vi "LakeShore 370 curve.vi"(2 "error in (no error)":errorcluster, 3 "Curve Data Format 1: Log Ohms/K)":u16(ring)=1 items=["Ohms/K", "Log Ohms/K"], 4 "Curve (1)":i32=1 min=1 max=20 step=1, 5 "VISA session":refnum<visa-resource-name>) -> (0 "error out":errorcluster, 1 "dup VISA session":refnum<visa-resource-name>)   [LabVIEW 2019]
doc: "This VI will upload a calibration curve to the LakeShore 370 AC Resistance Bridge. It reads the data from a file and then formats it for uploading.\nScott Hannahs, <sth@magnet.fsu.edu> NHMFL-FSU, May 2003"
uses:
  Misc Extras/Manufacturer Drivers/LakeShore/Lake Shore Cryotronics 370/Lake Shore Cryotronics 370.lvlib
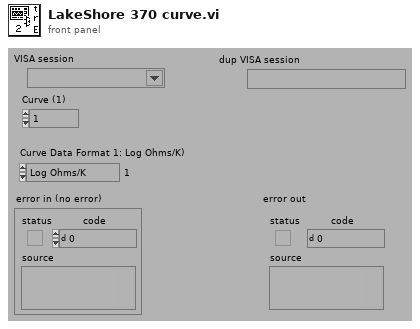
[diagram p1: front panel]
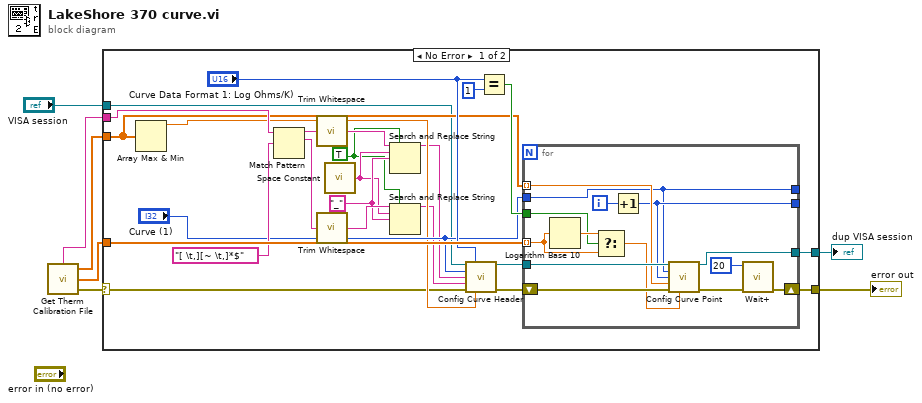
[diagram p0: block diagram]
diagram:
  n1 = call "Get Therm Calibration File.vi"() -> ("Calbration Name"=w6:string, "Temperature"=w5:dbl[], "Resistance"=w7:dbl[], "error out"=w1:errorcluster)  [unwired: 1 in]
  n2 = case shown="No Error" w1 {
    selector: w1 -> [w16 w46]
    tunnel: w7 -> [w31 _]
    tunnel: w6 -> [w24 _]
    tunnel: w5 -> [w21 _]
    tunnel: "VISA session" -> [w19 w47]
    tunnel: [w18 w46] -> w3
    tunnel: [w17 w47] -> w2
    frame No Error {
      w8 = TRUE ("replace all? (F)")
      w10 = "_" ("replace string (\"\")")
      n3 = Array Max & Min(array=w21) -> (max value=w20:dbl)  [unwired: 3 out]
      n4 = Match Pattern(string=w24, regular expression="[ \t,][~ \t,]*$") -> (before substring=w23:string, match substring=w15:string)  [unwired: 1 in, 2 out]
      n5 = call <vilib>:"Trim Whitespace.vi"("string"=w23) -> ("trimmed string"=w12:string)  [unwired: 1 in]
      n6 = call <vilib>:"Trim Whitespace.vi"("string"=w15) -> ("trimmed string"=w14:string)  [unwired: 1 in]
      n7 = call <vilib>:"Space Constant.vi"() -> ("String"=w9:string)
      n8 = Search and Replace String(replace all?=w8, input string=w12, search string=w9, replace string=w10) -> (result string=w11:string)  [unwired: 4 in, 3 out]
      n9 = Search and Replace String(replace all?=w8, input string=w14, search string=w9, replace string=w10) -> (result string=w13:string)  [unwired: 4 in, 3 out]
      n10 = call "Config Curve Header.vi"("VISA resource name"=w19, "Curve Data Format (0: Ohms/K)"="Curve Data Format 1: Log Ohms/K)", "Curve (1)"="Curve (1)", "Curve Name (\"\")"=w11, "Curve Serial Number (\"\")"=w13, "error in (no error)"=w16, "Limit Value (0.000)"=w20) -> ("VISA resource name out"=w30:refnum<visa-resource-name>, "error out"=w29:errorcluster)  [unwired: 7 in]
      n11 = Equal?(x="Curve Data Format 1: Log Ohms/K)", y=u16 1) -> (x = y?=w26:bool)
      n12 = for {
        tunnel: w21 -> [w43] mode=indexing
        tunnel: w31 -> [w39] mode=indexing
        tunnel: w30 -> [w45]
        tunnel: "Curve (1)" -> [w34]
        tunnel: w26 -> [w37]
        tunnel: [w36] -> w17
        tunnel: [w35] -> _
        tunnel: [w34] -> _
        shift-right: [w33] -> w18
        shift-left: w29 -> [w42]
        i -> [w44]
        n13 = Logarithm Base 10(1:w39) -> (0:w40:dbl)
        n14 = Select(t=w40, s=w37, f=w39) -> (s? t:f=w38:dbl)
        n15 = Increment(x=w44) -> (x+1=w35:i32)
        n16 = call "Config Curve Point.vi"("VISA resource name"=w45, "Curve (1)"=w34, "Index (1)"=w35, "Temperature Value (0.0000)"=w43, "error in (no error)"=w42, "Units Value (0.00000)"=w38) -> ("VISA resource name out"=w36:refnum<visa-resource-name>, "error out"=w41:errorcluster)  [unwired: 8 in]
        n17 = call "Wait+.vi"("Error In"=w41, "milliseconds to wait"=u32 20) -> ("Error Out"=w33:errorcluster)  [unwired: 4 in, 1 out]
      }
    }
    frame Error {
    }
  }
  "error out" <- w3
  "dup VISA session" <- w2
